vi "H5Dget_space_status.vi"(6 "error in (no error)":errorcluster, 9 "HDF5 Dataset Ref":T2) -> (0 "error out":errorcluster, 2 "Status":T1 items=["H5D_SPACE_STATUS_ERROR"=-1, "H5D_SPACE_STATUS_NOT_ALLOCATED"=0, "H5D_SPACE_STATUS_ALLOCATED"=1, "H5D_SPACE_STATUS_PART_ALLOCATED"=2], 3 "HDF5 Dataset Ref out":T2)   [LabVIEW 2017]
doc: "Determines whether space has been allocated for a dataset."
uses:
  <vilib>/UPVI/lvhdf5/library.llb/HDF5 Ref.ctl
  <vilib>/UPVI/lvhdf5/dataset.llb/H5D_space_status_t.ctl
  <vilib>/UPVI/lvhdf5/hdf5.dll
panel:
  # "LVHDF5 Toolkit\nCopyright (c) 2005-2013 by Jason D. Sommerville\nCopyright (c) 2014 by UPVI, LLC.\n\nThis use and distribution of this file is governed by the terms found in \nLICENSE.txt distributed with this toolkit and installed at\n <user.lib>\\_lvhdf5\\LICENSE.txt"
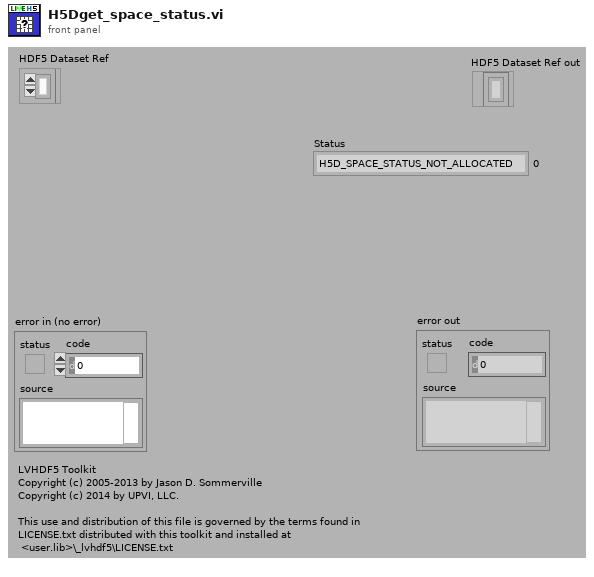
[diagram p1: front panel]
types:
  T1 = typedef "H5D_space_status_t.ctl" = i32
  T2 = typedef "HDF5 Ref.ctl" = refnum<k1>
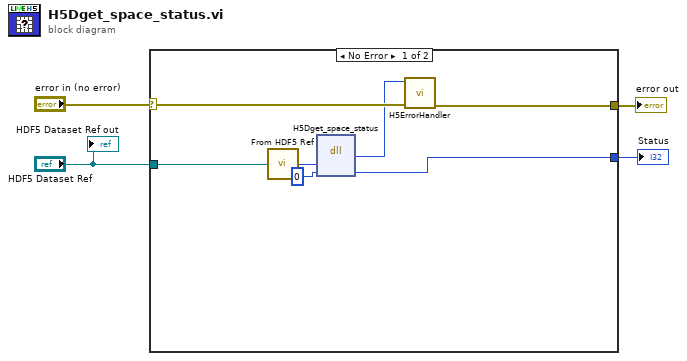
[diagram p0: block diagram]
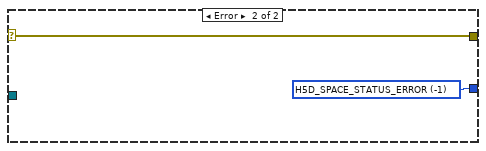
[diagram p2: hidden frame]
diagram:
  n1 = case shown="No Error" "error in (no error)" {
    selector: "error in (no error)" -> [w9 w13]
    tunnel: [w8 w13] -> w2
    tunnel: "HDF5 Dataset Ref" -> [w11 _]
    tunnel: [w5 w12] -> w1
    frame No Error {
      n2 = call <vilib>:"From HDF5 Ref.vi"("HDF5 Ref"=w11) -> ("I32"=w10:i32)
      n3 = dll-call lib="C:/Program Files/National Instruments/LabVIEW 2017/vi.lib/UPVI/lvhdf5/hdf5.dll" fn="H5Dget_space_status"("dset_id"=w10, "status"=0) -> (w7:i32, "status"=w5:i32)  [unwired: 4 in, 2 out]
      n4 = call <vilib>:"H5ErrorHandler.vi"("error in (no error)"=w9, "herr_t"=w7) -> ("error out"=w8:errorcluster)  [unwired: 3 in, 4 out]
    }
    frame Error {
      w12 = T1 -1 items=["H5D_SPACE_STATUS_ERROR"=-1, "H5D_SPACE_STATUS_NOT_ALLOCATED"=0, "H5D_SPACE_STATUS_ALLOCATED"=1, "H5D_SPACE_STATUS_PART_ALLOCATED"=2] ("Status")
    }
  }
  "error out" <- w2
  "Status" <- w1
  "HDF5 Dataset Ref out" <- "HDF5 Dataset Ref"
